vi "FM_Receiver_X32.vi"() -> ()   [LabVIEW 2013]
uses:
  <vilib>/sound2/lvsound2.llb/Sound Data Format.ctl
  <vilib>/Analysis/2dsp.llb/Decimate (single shot, DBL).vi
  <vilib>/Analysis/3filter.llb/Elliptic Filter (DBL).vi
  <vilib>/sound2/lvsound2.llb/Sound Output Write (DBL).vi
  <vilib>/Analysis/NI_AALBase.lvlib
  <vilib>/Analysis/NI_AALPro.lvlib
panel:
  out "error out 2":errorcluster
  in  "sound format":T1={"sample rate (S/s)"=44100.0, "number of channels"=2, "bits per sample"=16}
  in  "SampleFrequencyMHz":dbl=2.0 format="%#_13g"
  out "error out":errorcluster
  in  "reference":refnum<k24>
  in  "Device index":i32
  in  "CarrierFrequencyMHz":dbl=104.3
  out "Numeric":i32
  in  "stop":bool
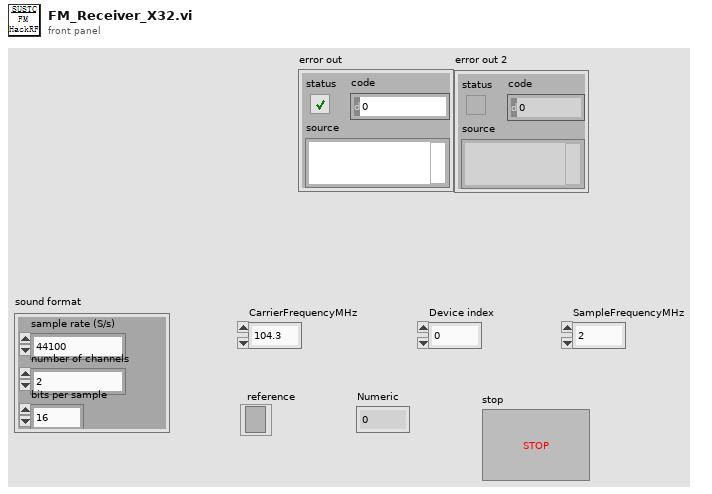
[diagram p1: front panel]
types:
  T1 = typedef "Sound Data Format.ctl" = cluster{"sample rate (S/s)":dbl, "number of channels":i32, "bits per sample":i32}
  T2 = typedef "Sound Output Task ID.ctl" = u32
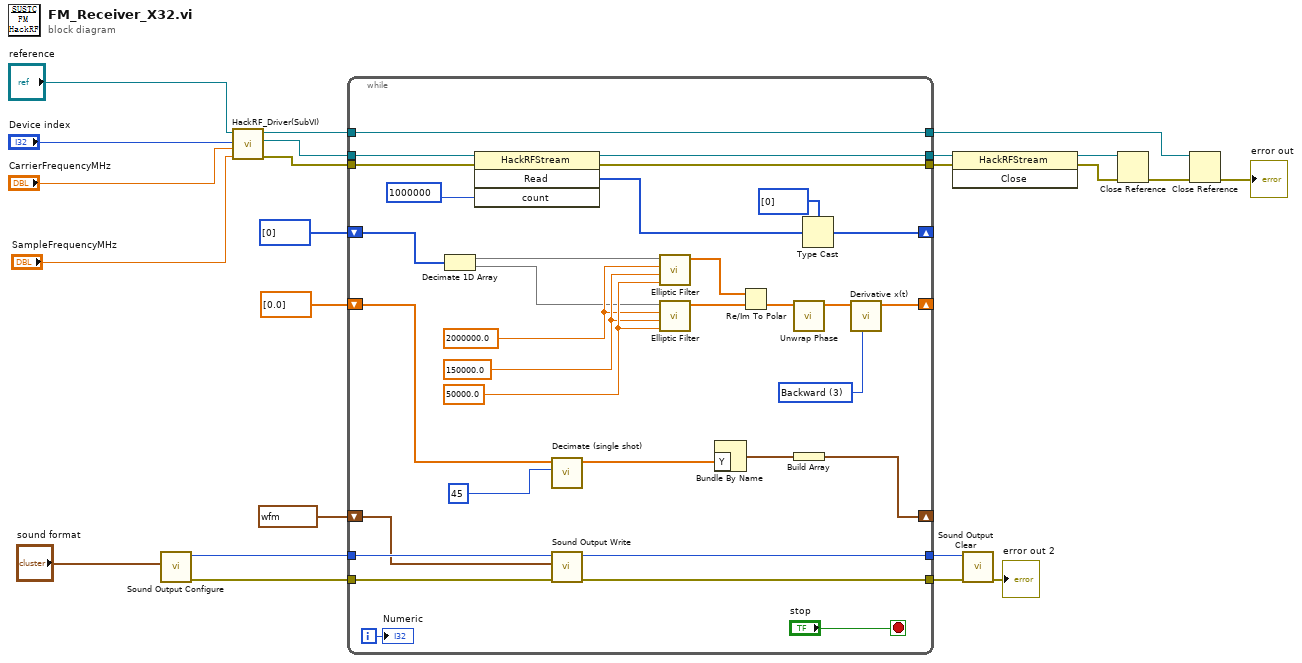
[diagram p0: block diagram]
diagram:
  n1 = call <vilib>:"Sound Output Configure.vi"("sound format"="sound format") -> ("error out"=w2:errorcluster, "task ID"=w3:T2)  [unwired: 9 in]
  n2 = call "HackRF_Driver(SubVI).vi"("SampleFrequencyMHz"="SampleFrequencyMHz", "CarrierFrequencyMHz"="CarrierFrequencyMHz", "Device index"="Device index", ".NET Refnum in"="reference") -> ("error out"=w12:errorcluster, "StartRX"=w13:refnum<k24>, ".NET Refnum out"=w23:refnum<k24>)  [unwired: 5 in]
  n3 = while {
    tunnel: w23 -> [w56]
    tunnel: [w56] -> w19
    tunnel: w3 -> [w53]
    tunnel: [w25] -> w18
    tunnel: [w24] -> w16
    tunnel: w2 -> [w50]
    tunnel: w13 -> [w49]
    tunnel: w12 -> [w48]
    tunnel: [w47] -> w11
    tunnel: [w46] -> w10
    shift-right: [w33] -> _
    shift-left: i8[] [0] ("Read") -> [w32]
    shift-right: [w31] -> _
    shift-left: dbl[] [0.0] ("dX/dt") -> [w27]
    shift-right: [w30] -> _
    shift-left: waveform(dbl)[] [{"t0"=timestamp(0 s since 1904-01-01), "dt"=1.0, "Y"=[0.0]}] -> [w29]
    i -> [w52]
    stop <- "stop" stop-if-true
    w44 = u16 3 items=["2nd Order Central", "4th Order Central", "Forward", "Backward"] ("method")
    w42 = 50000.0 ("low cutoff freq: fl")
    w41 = 150000.0 ("high cutoff freq: fh")
    w40 = 2000000.0 ("sampling freq: fs")
    n4 = Decimate 1D Array(w32) -> (w39:i8[], w37:i8[])
    n5 = invoke class="HackRFStream" method="Read"(reference=w49, error in=w48, "count"=1000000) -> (reference out=w47:refnum<k24>, error out=w46:errorcluster, "Read"=w34:u8[])  [unwired: 1 in, 1 out]
    n6 = call-poly <vilib>:"Decimate (single shot).vi"("decimating factor"=45, "X"=w27) -> ("Decimated Array"=w28:dbl[])  [unwired: 8 in, 1 out]
    n7 = call-poly <vilib>:"Sound Output Write.vi"("error in (no error)"=w50, "data"=w29, "task ID"=w53) -> ("error out"=w24:errorcluster, "task ID out"=w25:T2)  [unwired: 7 in]
    n8 = call-poly <vilib>:"Elliptic Filter.vi"("low cutoff freq: fl"=w42, "high cutoff freq: fh"=w41, "sampling freq: fs"=w40, "X"=w39) -> ("Filtered X"=w35:dbl[])  [unwired: 6 in, 1 out]
    n9 = call-poly <vilib>:"Elliptic Filter.vi"("low cutoff freq: fl"=w42, "high cutoff freq: fh"=w41, "sampling freq: fs"=w40, "X"=w37) -> ("Filtered X"=w38:dbl[])  [unwired: 6 in, 1 out]
    n10 = Bundle By Name("Y"=w28) -> (w54:waveform(dbl))  [unwired: 1 in]
    n11 = Re/Im To Polar(2:w38, 3:w35) -> (0:w45:dbl[])  [unwired: 1 out]
    n12 = call <vilib>:"Unwrap Phase.vi"("Phase"=w45) -> ("Unwrapped Phase"=w43:dbl[])  [unwired: 9 in, 1 out]
    n13 = Build Array(w54) -> (w30:waveform(dbl)[])
    n14 = Type Cast(type=i8[] [0] ("Read"), x=w34) -> (*(type *) &x=w33:i8[])
    n15 = call <vilib>:"Derivative x(t).vi"("method"=w44, "X"=w43) -> ("dX/dt"=w31:dbl[])  [unwired: 8 in, 1 out]
    "Numeric" <- w52
  }
  n16 = invoke class="HackRFStream" method="Close"(reference=w11, error in=w10) -> (reference out=w22:refnum<k24>, error out=w21:errorcluster)  [unwired: 1 in, 1 out]
  n17 = call <vilib>:"Sound Output Clear.vi"("error in (no error)"=w16, "task ID"=w18) -> ("error out"=→"error out 2":errorcluster)  [unwired: 9 in]
  n18 = Close Reference(reference=w22, error in (no error)=w21) -> (error out=w20:errorcluster)
  n19 = Close Reference(reference=w19, error in (no error)=w20) -> (error out=→"error out":errorcluster)
